vi "Prepare Response.vi"(8 "error in (no error)":errorcluster, 11 "PINGREQ in":refnum<class "PINGREQ.lvclass">) -> (0 "error out":errorcluster, 1 "response prepared?":bool, 2 "ControlPacket response":refnum<class "ControlPacket.lvclass">, 3 "PINGREQ out":refnum<class "PINGREQ.lvclass">)   [LabVIEW 2013, in "MQTT_Control_Packets.lvlib" / "PINGREQ.lvclass"]
uses:
  PINGREQ.lvclass
  ControlPacket/ControlPacket.lvclass
  ControlPacket/ControlPacket.lvclass/ControlPacket.ctl
  PINGRESP/PINGRESP.lvclass
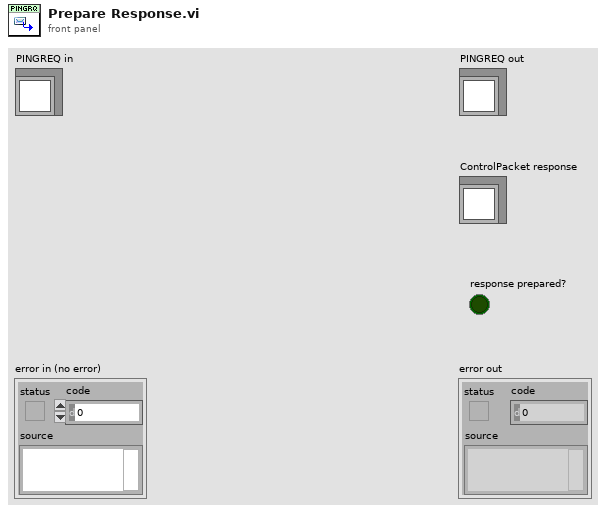
[diagram p1: front panel]
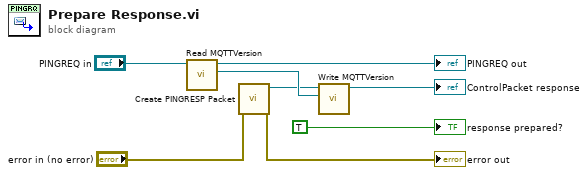
[diagram p0: block diagram]
diagram:
  n1 = call "Read MQTTVersion.vi"("ControlPacket in"="PINGREQ in") -> ("MQTTVersion"=w7:refnum<class "MQTTVersion.lvclass">, "ControlPacket out"=→"PINGREQ out":refnum<class "PINGREQ.lvclass">)  [unwired: 9 in]
  n2 = call "Create PINGRESP Packet.vi"("error in (no error)"="error in (no error)") -> ("error out"=→"error out":errorcluster, "PINGRESP out"=w6:refnum<class "PINGRESP.lvclass">)  [unwired: 8 in, 1 out]
  n3 = call "Write MQTTVersion.vi"("MQTTVersion"=w7, "ControlPacket in"=w6) -> ("ControlPacket out"=→"ControlPacket response":refnum<class "PINGRESP.lvclass">)  [unwired: 9 in]
  "response prepared?" <- TRUE ("response prepared?")
